vi "Write CEID.vi"(8 "error in (no error)":errorcluster, 10 "CEID":u32, 11 "07-Event Report From Equipment in":refnum<class "07-Event Report From Equipment.lvclass">) -> (0 "error out":errorcluster, 3 "07-Event Report From Equipment out":refnum<class "07-Event Report From Equipment.lvclass">)   [LabVIEW 2020, in "SECS Scenarios.lvlib" / "07-Event Report From Equipment.lvclass"]
uses:
  07-Event Report From Equipment.lvclass
  07-Event Report From Equipment.lvclass/07-Event Report From Equipment.ctl
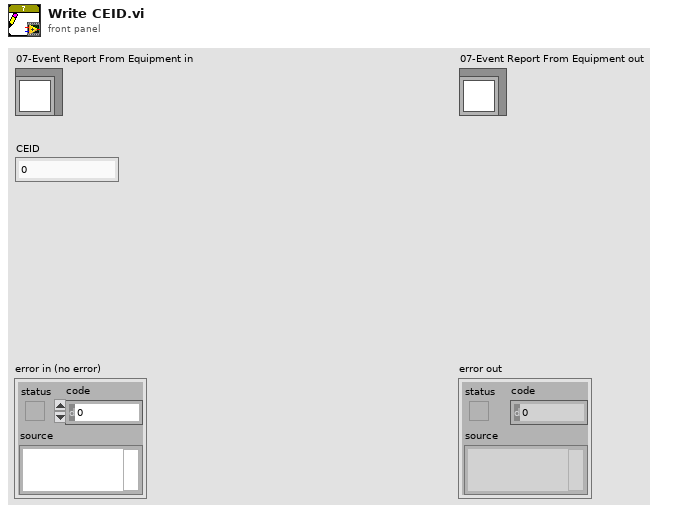
[diagram p1: front panel]
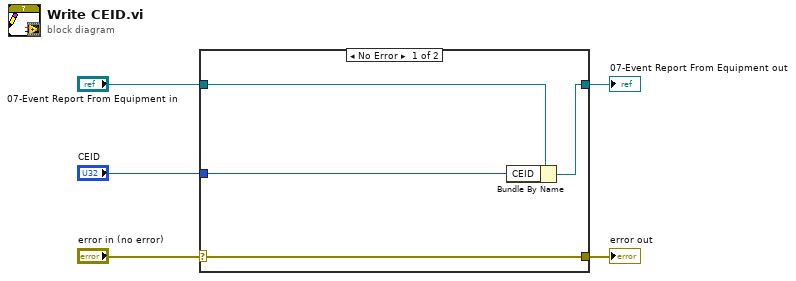
[diagram p0: block diagram]
diagram:
  n1 = case shown="No Error" "error in (no error)" {
    selector: "error in (no error)" -> [w9 w10]
    tunnel: [w9 w10] -> w4
    tunnel: [w7 w11] -> w2
    tunnel: "07-Event Report From Equipment in" -> [w8 w11]
    tunnel: "CEID" -> [w6 _]
    frame No Error {
      n2 = Bundle By Name(cluster=w8, "CEID"=w6) -> (w7:refnum<class "07-Event Report From Equipment.lvclass">)
    }
    frame Error {
    }
  }
  "error out" <- w4
  "07-Event Report From Equipment out" <- w2
